vi "Send Synchronous Message.vi"(7 "Message Priority (Normal)":T1=enum."Normal", 9 "Reply timeout in ms (-1)":i32, 10 "Message Enqueuer":refnum<class "Message Enqueuer.lvclass">, 11 "SynchronousMsg In":refnum<class "SynchronousMsg.lvclass">) -> (0 "error out":errorcluster, 2 "Actor Return Error":errorcluster, 3 "Data":variant)   [LabVIEW 2015, in "AbstractMessages.lvlib" / "SynchronousMsg.lvclass"]
doc: "<License>\nCopyright © 2017 Composed Systems, LLC | All rights reserved\nwww.composed.io\n\nAuthor: Ethan Stern <ethan.stern@composed.io>\n\nThis software is provided \"AS IS\" WITHOUT WARRANTIES, either express or implied, AND IS FOR EDUCATIONAL PURPOSES ONLY.\n</License>"
uses:
  SynchronousMsg.lvclass
  <vilib>/ActorFramework/Message Enqueuer/Message Enqueuer.lvclass
  <vilib>/ActorFramework/Message Enqueuer/Message Priority.ctl
  SynchronousMsg.lvclass/SynchronousMsg.ctl
  <vilib>/ActorFramework/Message Enqueuer/Message Enqueuer.lvclass/Message Enqueuer.ctl
  <vilib>/ActorFramework/Message Priority Queue/Priority Enqueue.vi
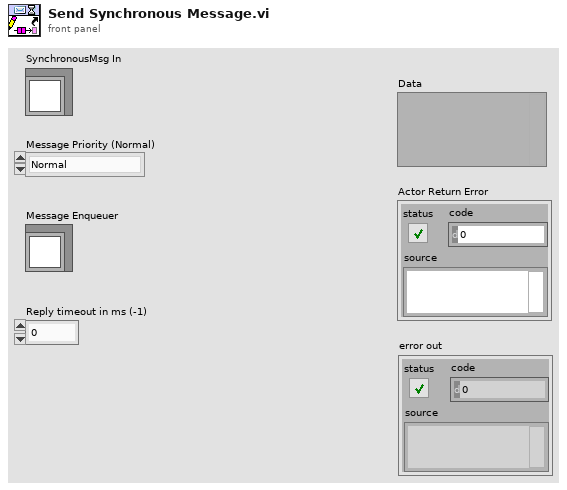
[diagram p1: front panel]
types:
  T1 = typedef "Actor Framework.lvlib/Message Enqueuer.lvclass/Message Priority.ctl" = enum16{"Low", "Normal", "High"}
  T2 = cluster{"Data":variant, "Return Error":errorcluster}
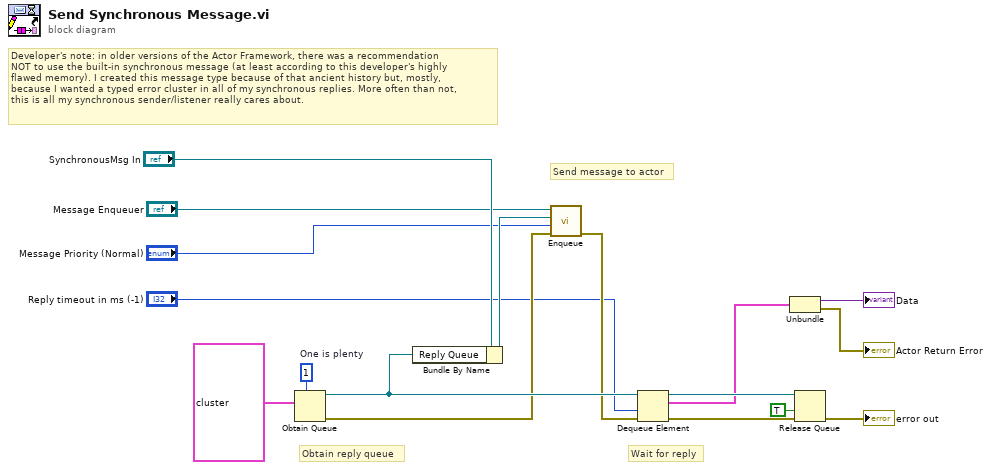
[diagram p0: block diagram]
diagram:
  w14 = 1  # One is plenty
  # "Obtain reply queue"
  # "Wait for reply"
  # "Send message to actor"
  # "Developer's note: in older versions of the Actor Framework, there was a recommendation\nNOT to use the built-in synchronous message (at least according to this developer's highly\nflawed memory). I created this message type because of that ancient history but, mostly, \nbecause I wanted a typed error cluster in all of my synchronous replies. More often than not,\nthis is all my synchronous sender/listener really cares about."
  n1 = Obtain Queue(max queue size (-1, unlimited)=w14, element data type=T2 {"Data"=variant, "Return Error"={"status"=FALSE, "code"=0, "source"=""}}) -> (queue out=w17:refnum<queue>, error out=w12:errorcluster)  [unwired: 3 in, 1 out]
  n2 = Bundle By Name(cluster="SynchronousMsg In", "Reply Queue"=w17) -> (w11:refnum<class "SynchronousMsg.lvclass">)
  n3 = call <vilib>:"Enqueue.vi"("error in (no error)"=w12, "Message Priority (Normal)"="Message Priority (Normal)", "Message"=w11, "Message Enqueuer in"="Message Enqueuer") -> ("error out"=w9:errorcluster)  [unwired: 6 in, 1 out]
  n4 = Dequeue Element(queue=w17, timeout in ms (-1)="Reply timeout in ms (-1)", error in (no error)=w9) -> (queue out=w8:refnum<queue>, element=w3:T2, error out=w7:errorcluster)  [unwired: 1 out]
  n5 = Unbundle(w3) -> ("Data"=→"Data":variant, "Return Error"=→"Actor Return Error":errorcluster)
  n6 = Release Queue(queue=w8, force destroy? (F)=TRUE, error in (no error)=w7) -> (error out=→"error out":errorcluster)  [unwired: 2 out]
